vi "buscar instrumentos.vi"() -> ()   [LabVIEW 2009]
uses:
  icon/nuevos/Control 20.ctl
panel:
  out "Numeric 3":i32
  out "Numeric 2":i32
  out "Numeric":i32
  out "Tab Control 2":T1
  out "Tab Control":T2(tab)
  out "Slide":i32(slide) scale=0.0..100.0
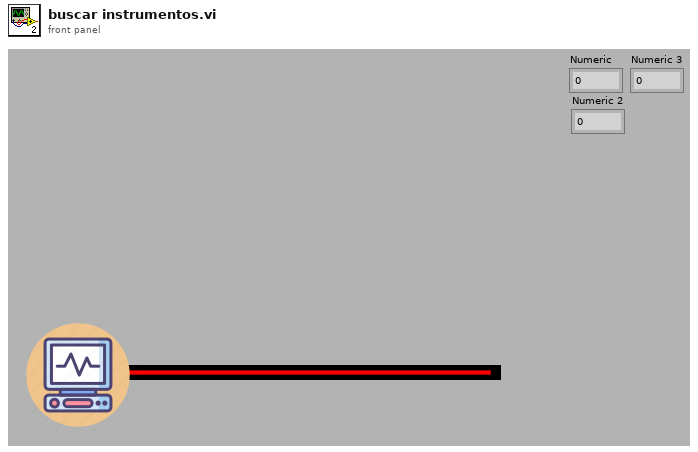
[diagram p1: front panel]
types:
  T1 = typedef "Control 20.ctl" = enum32{"Fuente", "Usb", "cta", "Polimetro", "Cpu", "apreton", "Alerta", "chip", "Calcula", "danger", "monitor", "Semaforo", "reset", "stop", "power", "info", "Enchufe", "Board", "Generator", "Oscilo"}
  T2 = enum32{"Fuente", "Usb", "cta", "Polimetro", "Cpu", "apreton", "Alerta", "chip", "Calcula", "danger", "monitor", "Semaforo", "reset", "stop", "power", "info", "Enchufe", "Board", "Generator", "Oscilo"}
  T3 = cluster{"OPCION":enum16{"animacion", "salir"}, "salir":bool}
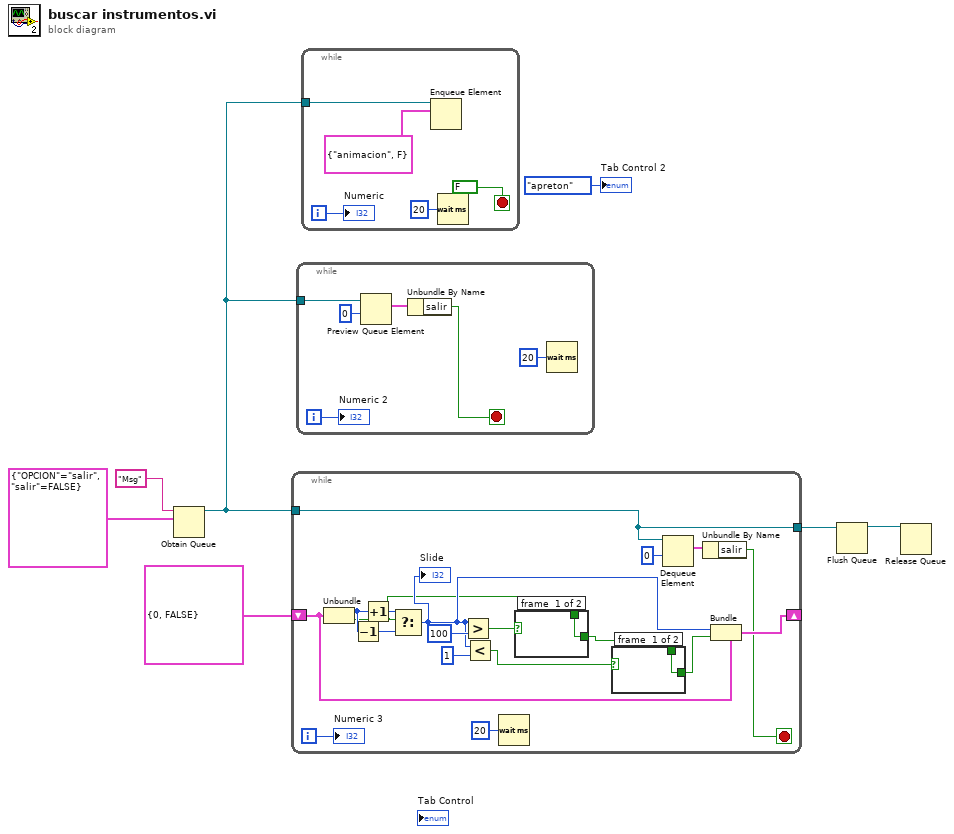
[diagram p0: block diagram]
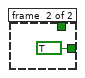
[diagram p2: hidden frame]
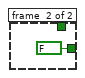
[diagram p3: hidden frame]
diagram:
  n1 = Obtain Queue(name (unnamed)="Msg", element data type=T3 {"OPCION"=enum."salir", "salir"=FALSE}) -> (queue out=w3:refnum<queue>)  [unwired: 3 in, 2 out]
  n2 = while {
    tunnel: w3 -> [w10]
    shift-right: [w13] -> _
    shift-left: cluster{i32, bool} {0, FALSE} -> [w22]
    tunnel: [w10] -> w2
    i -> [w9]
    stop <- w12 stop-if-true
    n3 = Unbundle(w22) -> (w25:i32, w16:bool)
    n4 = Decrement(x=w25) -> (x-1=w24:i32)
    n5 = Increment(x=w25) -> (x+1=w26:i32)
    n6 = Select(t=w26, s=w16, f=w24) -> (s? t:f=w20:i32)
    "Slide" <- w20
    n7 = Greater?(x=w20, y=100) -> (0:w18:bool)
    n8 = Less?(x=w20, y=1) -> (x < y?=w17:bool)
    n9 = Wait (ms)(milliseconds to wait=u32 20) -> ()  [unwired: 1 out]
    n10 = case shown="False" w18 {
      tunnel: [w29 FALSE] -> w15
      tunnel: w16 -> [w29 _]
      frame #0 {
      }
      frame #1 {
      }
    }
    n11 = case shown="True" w17 {
      tunnel: [w27 TRUE] -> w14
      tunnel: w15 -> [w27 _]
      frame #0 {
      }
      frame #1 {
      }
    }
    n12 = Dequeue Element(queue=w10, timeout in ms (-1)=0) -> (element=w11:T3)  [unwired: 1 in, 3 out]
    n13 = Unbundle By Name(w11) -> ("salir"=w12:bool)
    n14 = Bundle(cluster=w22, w20, w14) -> (w13:cluster{i32, bool})
    "Numeric 3" <- w9
  }
  n15 = while {
    tunnel: w3 -> [w36]
    i -> [w32]
    stop <- w34 stop-if-true
    n16 = Preview Queue Element(queue=w36, timeout in ms (-1)=0) -> (element=w35:T3)  [unwired: 1 in, 3 out]
    n17 = Unbundle By Name(w35) -> ("salir"=w34:bool)
    n18 = Wait (ms)(milliseconds to wait=u32 20) -> ()  [unwired: 1 out]
    "Numeric 2" <- w32
  }
  n19 = while {
    tunnel: w3 -> [w38]
    i -> [w39]
    stop <- FALSE stop-if-true
    n20 = Enqueue Element(queue=w38, element=T3 {"OPCION"=enum."animacion", "salir"=FALSE}) -> ()  [unwired: 2 in, 3 out]
    n21 = Wait (ms)(milliseconds to wait=u32 20) -> ()  [unwired: 1 out]
    "Numeric" <- w39
  }
  n22 = Flush Queue(queue=w2) -> (queue out=w1:refnum<queue>)  [unwired: 1 in, 2 out]
  n23 = Release Queue(queue=w1) -> ()  [unwired: 2 in, 3 out]
  "Tab Control 2" <- Control_20."apreton" ("Tab Control 2")
